vi "Plot_Server_Data.vi"() -> ()   [LabVIEW 2016]
uses:
  Anemometry/Anemometry Sub Vis/Controls/Server_Comms.ctl
  Anemometry/Anemometry Sub Vis/File/Setup_Filetype.ctl
  Anemometry/Anemometry Sub Vis/Globals/Preference_global.vi
panel:
  out "LastUpdated":string="Tue, May 12, 2015 at 11:28"
  in  "Throwback\n(mins)":dbl format="%.1f"
  in  "stop":bool=TRUE
  in  "Mode":T1(ring)=enum."Display data over specified period:"
  in  "History\n(mins)":dbl=20.0 format="%.1f"
  in  "Save plot number":T2(ring)
  out "Plot 3 Chs":string[](array[string])
  out "Plot 2 Chs":string[](array[string])
  out "Plot 1 Chs":string[](array[string])
  in  "Selector 1":i32[](listbox)
  in  "Search 1":string caption="Search:"
  in  "Search 2":string caption="Search:"
  in  "Search 3":string caption="Search:"
  in  "Selector 3":i32[](listbox)
  in  "Selector 2":i32[](listbox)
  in  "Precision":i32=2
  in  "Save 3":bool
  in  "palette3":i32(ring)=5 caption="Palette" items=["Strong", "Dark", "Light", "Pastel", "Pale", "Brash", "Clean", "Tidy"]
  out "Plot 3":cluster{"Times":dbl[], "Output array":dbl[]}[](graph)
  in  "Save 2":bool
  in  "palette2":i32(ring)=5 caption="Palette" items=["Strong", "Dark", "Light", "Pastel", "Pale", "Brash", "Clean", "Tidy"]
  out "Plot 2":cluster{"Times":dbl[], "Output array":dbl[]}[](graph)
  in  "Save 1":bool
  in  "palette1":i32(ring)=5 caption="Palette" items=["Strong", "Dark", "Light", "Pastel", "Pale", "Brash", "Clean", "Tidy"]
  out "Plot 1":cluster{"Times":dbl[], "Output array":dbl[]}[](graph)
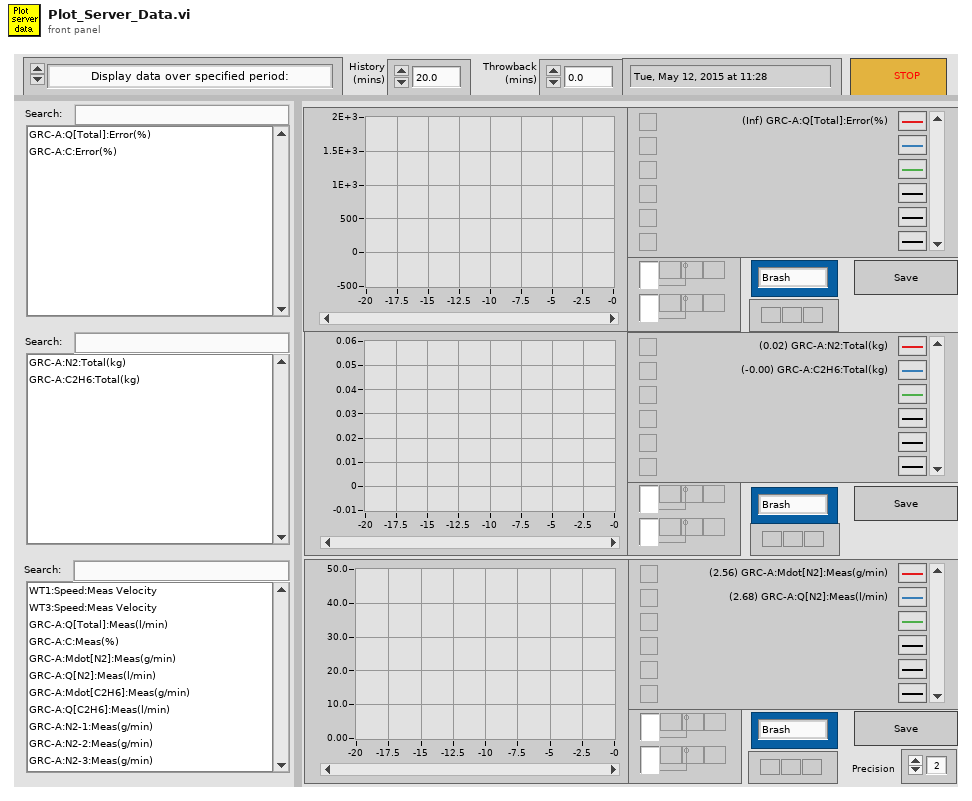
[diagram p1: front panel]
types:
  T1 = enum16{"Display full time history", "Display data over specified period:"}
  T2 = enum16{"Save Plot 1", "Save Plot 2", "Save Plot 3"}
  T3 = typedef "Server_Comms.ctl" = enum16{"Server Link Healthy", "Do Not Link To Server"}
  T4 = typedef "Setup_Filetype.ctl" = enum16{"Measurement Setups", "Calibration Setups", "General", "Results File Plotter Setups", "Speed Calib Tweaks"}
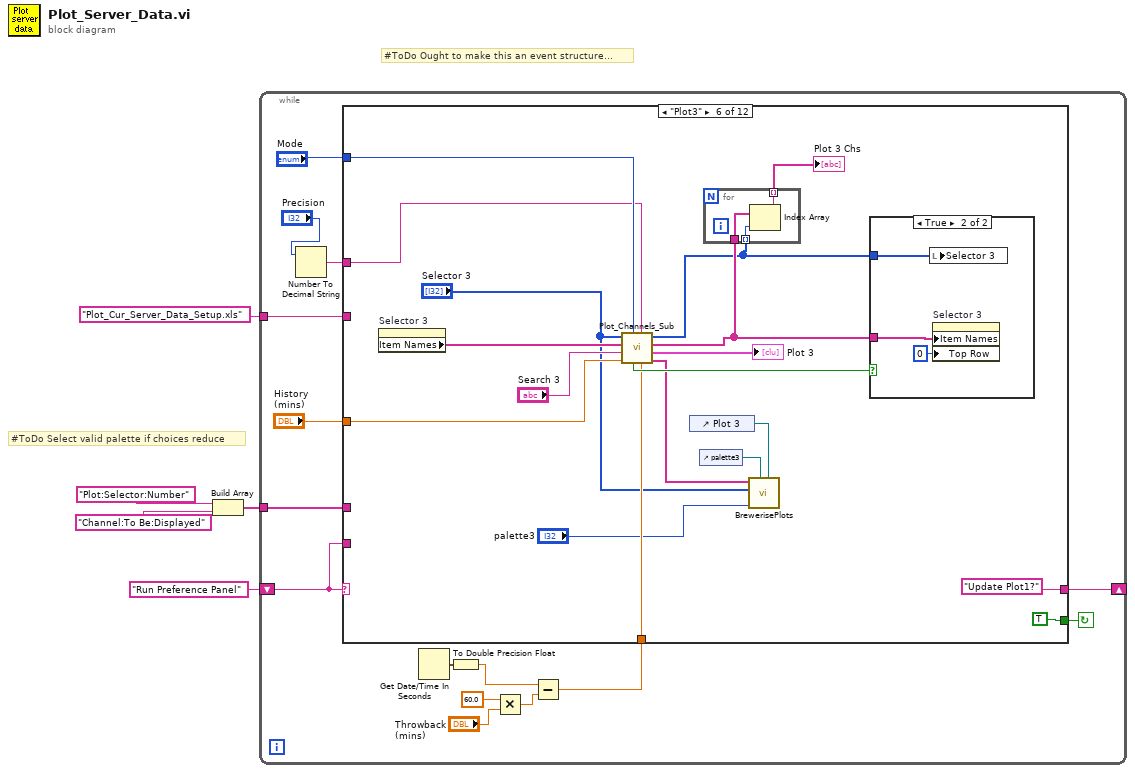
[diagram p0: block diagram]
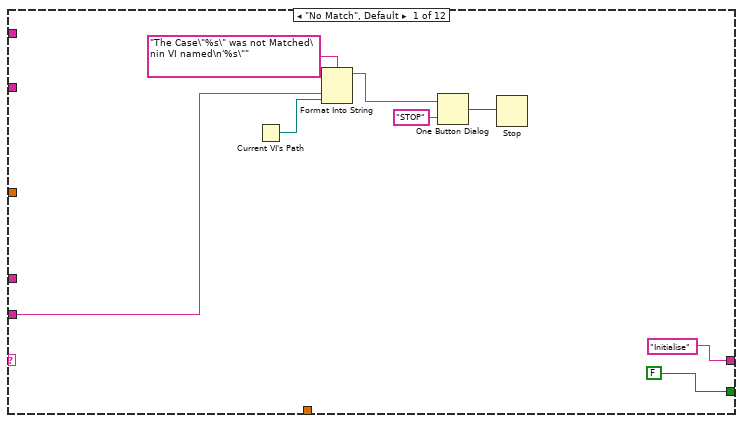
[diagram p2: hidden frame]
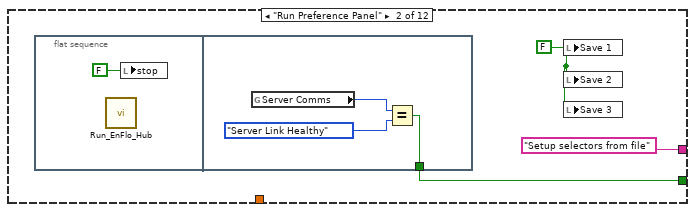
[diagram p3: hidden frame]
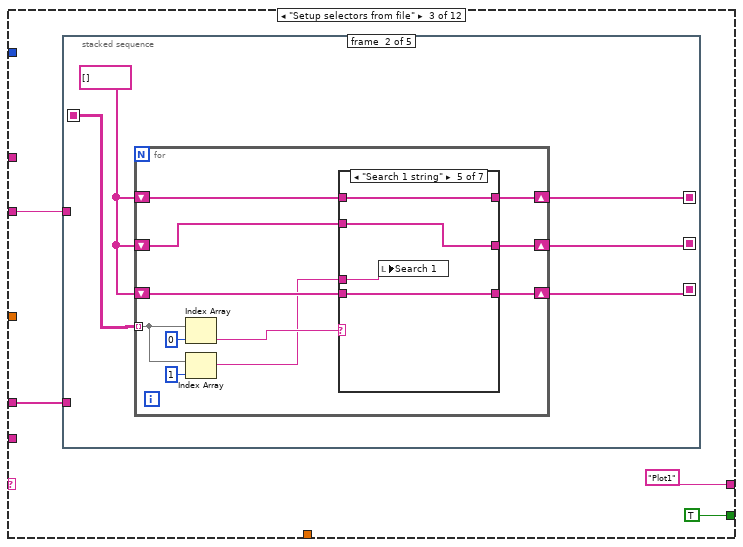
[diagram p4: hidden frame]
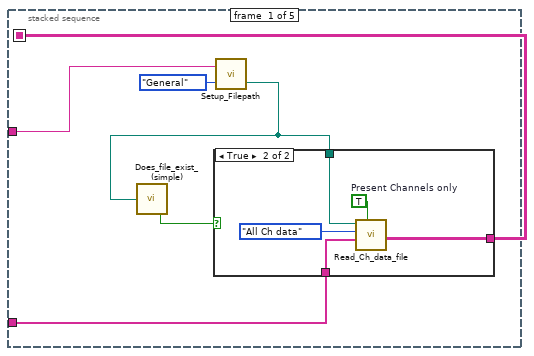
[diagram p5: hidden frame]
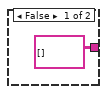
[diagram p6: hidden frame]
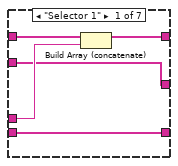
[diagram p7: hidden frame]
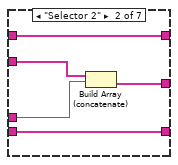
[diagram p8: hidden frame]
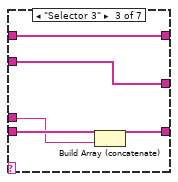
[diagram p9: hidden frame]
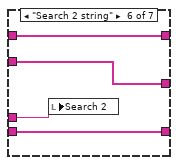
[diagram p11: hidden frame]
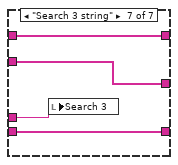
[diagram p12: hidden frame]
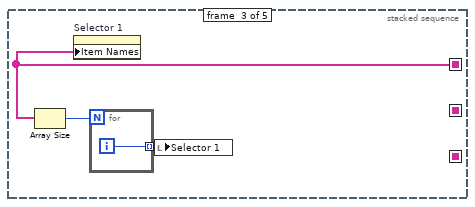
[diagram p13: hidden frame]
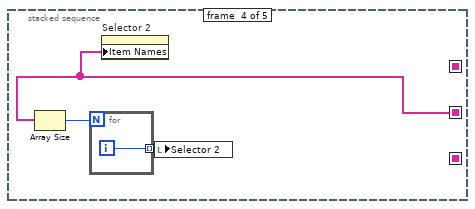
[diagram p14: hidden frame]
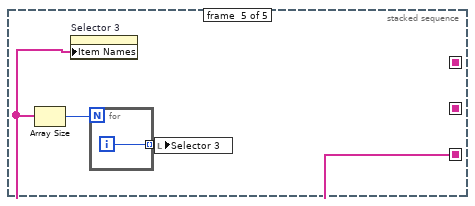
[diagram p15: hidden frame]
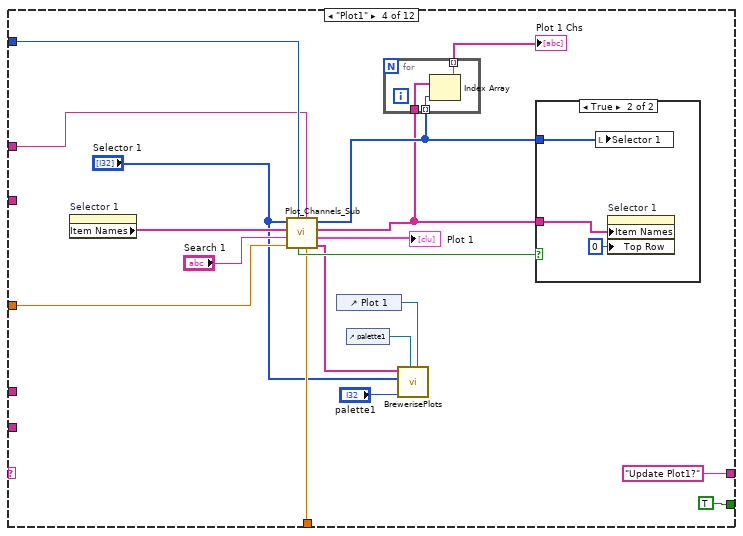
[diagram p16: hidden frame]
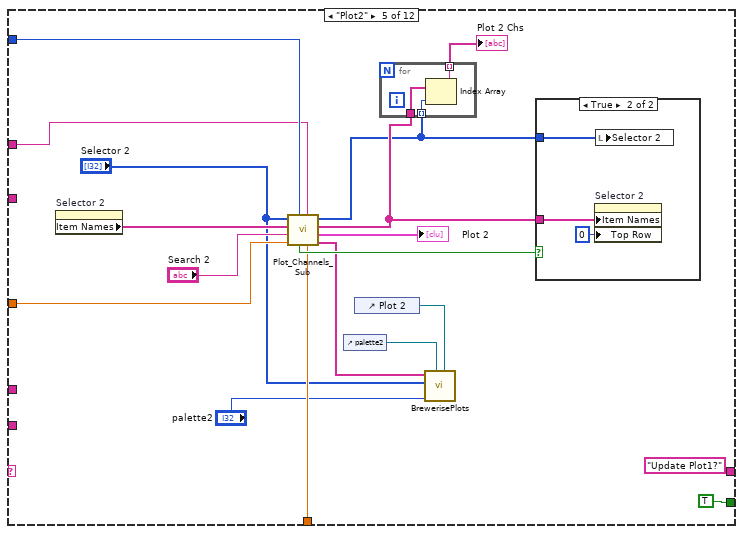
[diagram p18: hidden frame]
diagram:
  # "#ToDo Select valid palette if choices reduce"
  # "#ToDo Ought to make this an event structure..."
  n1 = Build Array("Plot:Selector:Number", "Channel:To Be:Displayed") -> (w2:string[])
  n2 = while {
    shift-left: "Run Preference Panel" -> [w18]
    shift-right: [w19] -> _
    tunnel: w2 -> [w15]
    tunnel: "Plot_Cur_Server_Data_Setup.xls" -> [w14]
    stop <- w20 continue-if-true
    n3 = Number To Decimal String(number="Precision") -> (decimal integer string=w12:string)  [unwired: 1 out]
    n4 = Get Date/Time In Seconds() -> (seconds since 1Jan1904=w11:timestamp)
    n5 = To Double Precision Float(number=w11) -> (double precision float=w7:dbl)
    n6 = Multiply(x=60.0, y="Throwback\n(mins)") -> (x*y=w8:dbl)
    n7 = Subtract(x=w7, y=w8) -> (x-y=w6:dbl)
    n8 = case shown="\"Plot3\"" w18 {
      tunnel: [FALSE w30 TRUE TRUE TRUE TRUE TRUE TRUE TRUE TRUE w323 w388] -> w20
      tunnel: ["Initialise" "Setup selectors from file" "Plot1" "Update Plot1?" "Update Plot1?" "Update Plot1?" w186 w212 w237 w271 w324 "Update Plot1?" ("t")] -> w19
      tunnel: w18 -> [w23 _ _ _ _ _ _ _ _ _ _ _]
      tunnel: "Mode" -> [_ _ _ w121 w148 w172 _ _ _ _ _ _]
      tunnel: "History\n(mins)" -> [_ _ _ w120 w147 w171 _ _ _ _ _ _]
      tunnel: w15 -> [_ _ w36 _ _ _ _ _ _ _ _ w392]
      tunnel: w14 -> [_ _ w37 _ _ _ _ _ _ _ _ w391]
      tunnel: w12 -> [_ _ _ w116 w140 w164 _ _ _ _ _ _]
      tunnel: w6 -> [_ _ _ w115 w139 w163 _ _ _ _ _ _]
      frame "No Match", Default {
        n9 = Current VI's Path() -> (path=w22:path)
        n10 = Format Into String(format string="The Case\"%s\" was not Matched\nin VI named\n'%s\"" ("Format String"), w23, w22) -> (resulting string=w26:string)  [unwired: 2 in, 1 out]
        n11 = One Button Dialog(message=w26, button name ("OK")="STOP") -> (true=w24:bool)
        n12 = Stop(stop? (T)=w24) -> ()
      }
      frame "Run Preference Panel" {
        w29 = FALSE ("Save 1")
        n13 = flat-sequence {
          tunnel: [w33] -> w30
          frame #0 {
            n14 = call "Run_EnFlo_Hub.vi"() -> ()  [unwired: 1 in, 7 out]
            n15 = local write "stop"(FALSE ("stop")) -> ()
          }
          frame #1 {
            n16 = global read "Preference_global.vi" "Server Comms"() -> (w34:T3)
            n17 = Equal?(x=w34, y=Server_Comms."Server Link Healthy" ("Server Comms")) -> (x = y?=w33:bool)
          }
        }
        n18 = local write "Save 1"(w29) -> ()
        n19 = local write "Save 2"(w29) -> ()
        n20 = local write "Save 3"(w29) -> ()
      }
      frame "Setup selectors from file" {
        n21 = stacked-sequence {
          seq-local: [w43 _ _ _ _] -> [_ w56 _ _ _]
          seq-local: [_ w54 _ _ _] -> [_ _ w100 _ _]
          seq-local: [_ w52 _ _ _] -> [_ _ _ w102 _]
          seq-local: [_ w53 _ _ _] -> [_ _ _ _ w106]
          tunnel: w37 -> [w42 _ _ _ _]
          tunnel: w36 -> [w44 _ _ _ _]
          frame #0 {
            n22 = call "Setup_Filepath.vi"("Setup File Type"=Setup_Filetype."General", "Filename in"=w42) -> ("Filename Out"=w41:path)  [unwired: 1 out]
            n23 = call "Does_file_exist_(simple).vi"("Pathname"=w41) -> ("exists?"=w45:bool)
            n24 = case shown="True" w45 {
              tunnel: w41 -> [_ w51]
              tunnel: w44 -> [_ w50]
              tunnel: [string[][] [] ("Channel Values") w47] -> w43
              frame False {
              }
              frame True {
                w49 = TRUE  # Present Channels only
                n25 = call "Read_Ch_data_file.vi"("Present Channels only"=w49, "Present Channels"=w50, "Output"=enum16{"All Ch data", "The last few rows"}."All Ch data", "Filename"=w51) -> ("Channel Values"=w47:string[][])  [unwired: 1 in, 4 out]
              }
            }
          }
          frame #1 {
            w55 = string[] []
            n26 = for {
              shift-right: [w62] -> w54
              shift-left: w55 -> [w63]
              tunnel: w56 -> [w64] mode=indexing
              shift-right: [w60] -> w52
              shift-left: w55 -> [w61]
              shift-right: [w58] -> w53
              shift-left: w55 -> [w59]
              n27 = Index Array(array=w64, index=0 ("Index")) -> (element=w66:string)
              n28 = Index Array(array=w64, index=1 ("Index")) -> (element=w57:string)
              n29 = case shown="\"Search 1 string\"" w66 {
                tunnel: w63 -> [w72 w77 w78 w84 w88 w92 w96]
                tunnel: [w71 w77 w78 w84 w88 w92 w96] -> w62
                tunnel: w57 -> [w70 w74 w80 _ w86 w90 w94]
                tunnel: w61 -> [w69 w75 w79 w85 w89 w93 w97]
                tunnel: [w69 w73 w79 w85 w89 w93 w97] -> w60
                tunnel: w59 -> [w68 w76 w82 w83 w87 w91 w95]
                tunnel: [w68 w76 w81 w83 w87 w91 w95] -> w58
                frame "Selector 1" {
                  n30 = Build Array (concatenate)(w72, w70) -> (w71:string[])
                }
                frame "Selector 2" {
                  n31 = Build Array (concatenate)(w75, w74) -> (w73:string[])
                }
                frame "Selector 3" {
                  n32 = Build Array (concatenate)(w82, w80) -> (w81:string[])
                }
                frame "No Match", Default {
                }
                frame "Search 1 string" {
                  n33 = local write "Search 1"(w86) -> ()
                }
                frame "Search 2 string" {
                  n34 = local write "Search 2"(w90) -> ()
                }
                frame "Search 3 string" {
                  n35 = local write "Search 3"(w94) -> ()
                }
              }
            }
          }
          frame #2 {
            n36 = Array Size(array=w100) -> (size(s)=w99:i32)
            n37 = property on="Selector 1" class="LstBox (strict)"("Item Names"=w100) -> ()  [unwired: 2 in, 2 out]
            n38 = for {
              N: w99 -> [_]
              tunnel: [w101] -> w98 mode=indexing
              i -> [w101]
            }
            n39 = local write "Selector 1"(w98) -> ()
          }
          frame #3 {
            n40 = Array Size(array=w102) -> (size(s)=w104:i32)
            n41 = for {
              N: w104 -> [_]
              tunnel: [w105] -> w103 mode=indexing
              i -> [w105]
            }
            n42 = property on="Selector 2" class="LstBox (strict)"("Item Names"=w102) -> ()  [unwired: 2 in, 2 out]
            n43 = local write "Selector 2"(w103) -> ()
          }
          frame #4 {
            n44 = Array Size(array=w106) -> (size(s)=w108:i32)
            n45 = property on="Selector 3" class="LstBox (strict)"("Item Names"=w106) -> ()  [unwired: 2 in, 2 out]
            n46 = for {
              N: w108 -> [_]
              tunnel: [w109] -> w107 mode=indexing
              i -> [w109]
            }
            n47 = local write "Selector 3"(w107) -> ()
          }
        }
      }
      frame "Plot1" {
        n48 = property on="Selector 1" class="LstBox (strict)"() -> ("Item Names"=w122:string[])  [unwired: 2 in, 2 out]
        n49 = call "Plot_Channels_Sub.vi"("End Time"=w115, "precision"=w116, "Mode"=w121, "History (min)"=w120, "Search String"="Search 1", "Selector List In"=w122, "Selector array In"="Selector 1") -> ("Plot Legend"=w112:string[], "Plot"=→"Plot 1":cluster{"Times":dbl[], "Output array":dbl[]}[], "Selector List Out"=w118:string[], "Selector array Out"=w119:i32[], "Selector Changed?"=w124:bool)
        n50 = control-ref of="Plot 1"() -> (w114:refnum<vi>)
        n51 = control-ref of="palette1"() -> (w113:refnum<vi>)
        n52 = for {
          tunnel: w119 -> [w130] mode=indexing
          tunnel: w118 -> [w129]
          tunnel: [w128] -> w117 mode=indexing
          n53 = Index Array(array=w129, index=w130) -> (element=w128:string)
        }
        "Plot 1 Chs" <- w117
        n54 = call "BrewerisePlots.vi"("graphRefnum"=w114, "paletteRefnum"=w113, "paletteNum"="palette1", "Series"="Selector 1", "Plot Legends"=w112) -> ()  [unwired: 7 in]
        n55 = case shown="True" w124 {
          tunnel: w118 -> [_ w133]
          tunnel: w119 -> [_ w132]
          frame False {
          }
          frame True {
            n56 = local write "Selector 1"(w132) -> ()
            n57 = property on="Selector 1" class="LstBox (strict)"("Item Names"=w133, "Top Row"=0) -> ()  [unwired: 2 in, 2 out]
          }
        }
      }
      frame "Plot2" {
        n58 = property on="Selector 2" class="LstBox (strict)"() -> ("Item Names"=w144:string[])  [unwired: 2 in, 2 out]
        n59 = call "Plot_Channels_Sub.vi"("End Time"=w139, "precision"=w140, "Mode"=w148, "History (min)"=w147, "Search String"="Search 2", "Selector List In"=w144, "Selector array In"="Selector 2") -> ("Plot Legend"=w136:string[], "Plot"=→"Plot 2":cluster{"Times":dbl[], "Output array":dbl[]}[], "Selector List Out"=w143:string[], "Selector array Out"=w142:i32[], "Selector Changed?"=w149:bool)
        n60 = control-ref of="palette2"() -> (w137:refnum<vi>)
        n61 = control-ref of="Plot 2"() -> (w138:refnum<vi>)
        n62 = for {
          tunnel: w142 -> [w154] mode=indexing
          tunnel: w143 -> [w153]
          tunnel: [w152] -> w141 mode=indexing
          n63 = Index Array(array=w153, index=w154) -> (element=w152:string)
        }
        "Plot 2 Chs" <- w141
        n64 = call "BrewerisePlots.vi"("graphRefnum"=w138, "paletteRefnum"=w137, "paletteNum"="palette2", "Series"="Selector 2", "Plot Legends"=w136) -> ()  [unwired: 7 in]
        n65 = case shown="True" w149 {
          tunnel: w143 -> [_ w156]
          tunnel: w142 -> [_ w157]
          frame False {
          }
          frame True {
            n66 = property on="Selector 2" class="LstBox (strict)"("Item Names"=w156, "Top Row"=0) -> ()  [unwired: 2 in, 2 out]
            n67 = local write "Selector 2"(w157) -> ()
          }
        }
      }
      frame "Plot3" {
        n68 = property on="Selector 3" class="LstBox (strict)"() -> ("Item Names"=w168:string[])  [unwired: 2 in, 2 out]
        n69 = call "Plot_Channels_Sub.vi"("End Time"=w163, "precision"=w164, "Mode"=w172, "History (min)"=w171, "Search String"="Search 3", "Selector List In"=w168, "Selector array In"="Selector 3") -> ("Plot Legend"=w160:string[], "Plot"=→"Plot 3":cluster{"Times":dbl[], "Output array":dbl[]}[], "Selector List Out"=w167:string[], "Selector array Out"=w166:i32[], "Selector Changed?"=w173:bool)
        n70 = control-ref of="Plot 3"() -> (w162:refnum<vi>)
        n71 = control-ref of="palette3"() -> (w161:refnum<vi>)
        n72 = for {
          tunnel: w166 -> [w178] mode=indexing
          tunnel: w167 -> [w177]
          tunnel: [w176] -> w165 mode=indexing
          n73 = Index Array(array=w177, index=w178) -> (element=w176:string)
        }
        "Plot 3 Chs" <- w165
        n74 = call "BrewerisePlots.vi"("graphRefnum"=w162, "paletteRefnum"=w161, "paletteNum"="palette3", "Series"="Selector 3", "Plot Legends"=w160) -> ()  [unwired: 7 in]
        n75 = case shown="True" w173 {
          tunnel: w167 -> [_ w180]
          tunnel: w166 -> [_ w181]
          frame False {
          }
          frame True {
            n76 = local write "Selector 3"(w181) -> ()
            n77 = property on="Selector 3" class="LstBox (strict)"("Item Names"=w180, "Top Row"=0) -> ()  [unwired: 2 in, 2 out]
          }
        }
      }
      frame "Update Plot1?" {
        n78 = while {
          shift-right: [w206] -> w193
          shift-left: _ -> [w203]
          shift-right: [w205] -> w195
          shift-left: _ -> [w204]
          tunnel: [w204] -> w194
          tunnel: [w203] -> w192
          shift-right: [w201] -> w183
          shift-left: _ -> [w200]
          tunnel: [w200] -> w184
          stop <- FALSE continue-if-true
          n79 = local read "Selector 1"() -> (w206:i32[])
          n80 = local read "palette1"() -> (w201:i32)
          n81 = local read "Search 1"() -> (w205:string)
        }
        n82 = case shown="False" "Save 1" {
          tunnel: ["Update Plot2?" "Save Plot" ("t")] -> w185
          frame False {
          }
          frame True {
            n83 = local write "Save plot number"(T2."Save Plot 1" ("Save plot number")) -> ()
          }
        }
        n84 = Equal?(x=w183, y=w184) -> (x = y?=w182:bool)
        n85 = Equal?(x=w193, y=w192) -> (x = y?=w190:bool)
        n86 = Equal?(x=w194, y=w195) -> (x = y?=w191:bool)
        n87 = Compound Arithmetic op=AND(w182, w190, w191) -> (w189:bool)
        n88 = Select(t=w185, s=w189, f="Plot1") -> (s? t:f=w186:string)
      }
      frame "Update Plot2?" {
        n89 = while {
          shift-right: [w231] -> w218
          shift-left: _ -> [w228]
          shift-right: [w230] -> w220
          shift-left: _ -> [w229]
          tunnel: [w229] -> w219
          tunnel: [w228] -> w217
          shift-right: [w226] -> w208
          shift-left: _ -> [w225]
          tunnel: [w225] -> w209
          stop <- FALSE continue-if-true
          n90 = local read "Selector 2"() -> (w231:i32[])
          n91 = local read "Search 2"() -> (w230:string)
          n92 = local read "palette2"() -> (w226:i32)
        }
        n93 = case shown="False" "Save 2" {
          tunnel: ["Update Plot3?" "Save Plot" ("t")] -> w210
          frame False {
          }
          frame True {
            n94 = local write "Save plot number"(T2."Save Plot 2" ("Save plot number")) -> ()
          }
        }
        n95 = Equal?(x=w208, y=w209) -> (x = y?=w207:bool)
        n96 = Equal?(x=w218, y=w217) -> (x = y?=w215:bool)
        n97 = Equal?(x=w219, y=w220) -> (x = y?=w216:bool)
        n98 = Compound Arithmetic op=AND(w207, w215, w216) -> (w214:bool)
        n99 = Select(t=w210, s=w214, f="Plot2") -> (s? t:f=w212:string)
      }
      frame "Update Plot3?" {
        n100 = while {
          shift-right: [w256] -> w243
          shift-left: _ -> [w253]
          shift-right: [w255] -> w245
          shift-left: _ -> [w254]
          tunnel: [w254] -> w244
          tunnel: [w253] -> w242
          shift-right: [w251] -> w234
          shift-left: _ -> [w250]
          tunnel: [w250] -> w233
          stop <- FALSE continue-if-true
          n101 = local read "Selector 3"() -> (w256:i32[])
          n102 = local read "Search 3"() -> (w255:string)
          n103 = local read "palette3"() -> (w251:i32)
        }
        n104 = case shown="False" "Save 3" {
          tunnel: ["What to do next?" "Save Plot" ("t")] -> w235
          frame False {
          }
          frame True {
            n105 = local write "Save plot number"(T2."Save Plot 3" ("Save plot number")) -> ()
          }
        }
        n106 = Equal?(x=w243, y=w242) -> (x = y?=w240:bool)
        n107 = Equal?(x=w244, y=w245) -> (x = y?=w241:bool)
        n108 = Equal?(x=w234, y=w233) -> (x = y?=w232:bool)
        n109 = Compound Arithmetic op=AND(w232, w240, w241) -> (w239:bool)
        n110 = Select(t=w235, s=w239, f="Plot3") -> (s? t:f=w237:string)
      }
      frame "What to do next?" {
        n111 = Wait (ms)(milliseconds to wait=u32 300) -> ()  [unwired: 1 out]
        n112 = while {
          shift-right: [w287] -> _
          shift-left: _ -> [w286]
          shift-right: [w285] -> _
          shift-left: _ -> [w284]
          shift-right: [w277] -> _
          shift-left: _ -> [w276]
          tunnel: [w279] -> w270
          shift-right: [w273] -> w259
          shift-left: _ -> [w274]
          stop <- FALSE continue-if-true
          n113 = local read "History\n(mins)"() -> (w287:dbl)
          n114 = local read "Mode"() -> (w285:T1)
          n115 = Equal?(x=w287, y=w286) -> (x = y?=w283:bool)
          n116 = Equal?(x=w284, y=w285) -> (x = y?=w282:bool)
          n117 = And(x=w283, y=w282) -> (x .and. y?=w281:bool)
          n118 = Select(t=w276, s=w281, f=0) -> (s? t:f=w278:i32)
          n119 = case shown="0, Default" w278 {
            tunnel: ["Plot1" "Plot2" "Plot3" "Update Plot1?" "Update Plot1?" "Update Plot1?" "Update Plot1?"] -> w279
            tunnel: w278 -> [w290 w294 w298 w304 w310 w316 _]
            tunnel: [w289 w293 w297 w303 w309 w315 0] -> w277
            tunnel: w274 -> [w288 w292 w296 w301 w307 w312 w319]
            tunnel: [w288 w292 w296 w300 w306 w313 w318] -> w273
            frame 0, Default {
              n120 = Increment(x=w290) -> (x+1=w289:i32)
            }
            frame 1 {
              n121 = Increment(x=w294) -> (x+1=w293:i32)
            }
            frame 2 {
              n122 = Increment(x=w298) -> (x+1=w297:i32)
            }
            frame 3 {
              n123 = Add(x=w301, y=1) -> (x+y=w300:i32)
              n124 = Increment(x=w304) -> (x+1=w303:i32)
            }
            frame 4 {
              n125 = Add(x=w307, y=1) -> (x+y=w306:i32)
              n126 = Increment(x=w310) -> (x+1=w309:i32)
            }
            frame 5 {
              n127 = Add(x=w312, y=1) -> (x+y=w313:i32)
              n128 = Increment(x=w316) -> (x+1=w315:i32)
            }
            frame 6 {
              n129 = Add(x=w319, y=1) -> (x+y=w318:i32)
            }
          }
        }
        n130 = Get Date/Time String(date format (0)=enum16{"short", "long", "abbreviated"}."abbreviated") -> (date string=w266:string, time string=w267:string)  [unwired: 2 out]
        n131 = Concatenate Strings(w266, " at " ("Substring"), w267) -> (→"LastUpdated":string)
        n132 = Quotient & Remainder(x=w259, y=500) -> (x-y*floor(x/y)=w263:i32)  [unwired: 1 out]
        n133 = Equal To 0?(x=w263) -> (x = 0?=w261:bool)
        n134 = Or(x="stop", y=w261) -> (x .or. y?=w260:bool)
        n135 = Select(t="Save Channel Names", s=w260, f=w270) -> (s? t:f=w271:string)
      }
      frame "Save Plot" {
        n136 = stacked-sequence {
          seq-local: [w335 _] -> [_ w363]
          seq-local: [w330 _] -> [_ w365]
          seq-local: [w334 _] -> [_ w364]
          seq-local: [w325 _] -> [_ w353]
          tunnel: ["What to do next?" _] -> w324
          tunnel: [TRUE _] -> w323
          frame #0 {
            n137 = case shown="\"Save Plot 1\"" "Save plot number" {
              tunnel: [w343 w346 w349] -> w340
              tunnel: [w342 w345 w348] -> w335
              frame "Save Plot 1" {
                n138 = local read "Plot 1 Chs"() -> (w342:string[])
                n139 = local write "Save 1"(FALSE ("Save 1")) -> ()
                n140 = local read "Plot 1"() -> (w343:cluster{"Times":dbl[], "Output array":dbl[]}[])
              }
              frame "Save Plot 2" {
                n141 = local read "Plot 2 Chs"() -> (w345:string[])
                n142 = local write "Save 2"(FALSE ("Save 1")) -> ()
                n143 = local read "Plot 2"() -> (w346:cluster{"Times":dbl[], "Output array":dbl[]}[])
              }
              frame "Save Plot 3" {
                n144 = local read "Plot 3 Chs"() -> (w348:string[])
                n145 = local write "Save 3"(FALSE ("Save 1")) -> ()
                n146 = local read "Plot 3"() -> (w349:cluster{"Times":dbl[], "Output array":dbl[]}[])
              }
            }
            n147 = Index Array(array=w340, index=0) -> (element=w338:cluster{"Times":dbl[], "Output array":dbl[]})
            n148 = Unbundle(w338) -> ("Times"=w329:dbl[])  [unwired: 1 out]
            n149 = Get Date/Time In Seconds() -> (seconds since 1Jan1904=w332:timestamp)
            n150 = for {
              tunnel: w340 -> [w351] mode=indexing
              tunnel: [w350] -> w334 mode=indexing
              n151 = Unbundle(w351) -> ("Output array"=w350:dbl[])  [unwired: 1 out]
            }
            n152 = To Double Precision Float(number=w332) -> (double precision float=w331:dbl)
            n153 = Multiply(x=w329, y=60.0) -> (x*y=w327:dbl[])
            n154 = Add(x=w331, y=w327) -> (x+y=w330:dbl[])
            n155 = Index Array(array=w327) -> (element=w326:dbl)  [unwired: 1 in]
            n156 = Subtract(x=w327, y=w326) -> (x-y=w325:dbl[])
          }
          frame #1 {
            w358 = FALSE  # append to file? (new file:F)
            n157 = for {
              tunnel: w364 -> [w385]
              tunnel: w365 -> [w379] mode=indexing
              tunnel: [w381] -> w357 mode=indexing
              tunnel: w353 -> [w375] mode=indexing
              i -> [w384]
              n158 = Number To Decimal String(number=w379) -> (decimal integer string=w380:string)  [unwired: 1 out]
              n159 = Index Array(array=w385, index (col)=w384) -> (element=w383:dbl[])  [unwired: 1 in]
              n160 = Number To Fractional String(number=w375, precision (6)=i16 2) -> (F-format string=w374:string)  [unwired: 2 in]
              n161 = Get Date/Time String(seconds (now)=w379) -> (date string=w378:string, time string=w377:string)  [unwired: 2 out]
              n162 = for {
                tunnel: w383 -> [w387] mode=indexing
                tunnel: [w386] -> w382 mode=indexing
                n163 = call "Number_2_string.vi"("number"=w387) -> ("String"=w386:string)  [unwired: 1 in]
              }
              n164 = Build Array (concatenate)(w378, w377, w380, w374, w382) -> (w381:string[])
            }
            n165 = Build Array (concatenate)("Date::", "Centre:Time:", "Seconds:Since:1st Jan 1904", "Time:in:Seconds", w363) -> (w356:string[])
            n166 = call "Ch_names_to_rows.vi"("Channel Names"=w356) -> ("3 Row names"=w362:string[][])
            n167 = File Dialog(7:"Please choose file name" ("prompt")) -> (3:w370:path)  [unwired: 1 in, 8 out]
            n168 = Build Array (concatenate)(w362, w357) -> (w360:string[][])
            n169 = Strip Path(path=w370) -> (stripped path=w367:path, name=w369:string)
            n170 = call "Add_filename_suffix.vi"("Filename"=w369, "Suffix to add"=".xls") -> ("Filename out"=w366:string)  [unwired: 3 out]
            n171 = Array To Spreadsheet String(array=w360, 3:"%s" ("format string")) -> (spreadsheet string=w359:string)  [unwired: 1 out]
            n172 = Build Path(base path=w367, name or relative path=w366) -> (appended path=w355:path)
            n173 = call "Write_File_Simple.vi"("append to file? (new file:F)"=w358, "character string"=w359, "file path"=w355) -> ()  [unwired: 2 out]
          }
        }
      }
      frame "Save Channel Names" {
        n174 = stacked-sequence {
          seq-local: [w394 _ _] -> [_ w418 _]
          seq-local: [_ w417 _] -> [_ _ w431]
          tunnel: w392 -> [_ _ w432]
          tunnel: w391 -> [_ _ w429]
          frame #0 {
            n175 = for {
              N: 3 -> [_]
              shift-right: [w398] -> w394
              shift-left: string[][] [] -> [w400]
              i -> [w405]
              n176 = Increment(x=w405) -> (x+1=w402:i32)
              n177 = case shown="1, Default" w402 {
                tunnel: [w412 w413 w415] -> w404
                tunnel: [w411 w414 w416] -> w396
                frame 1, Default {
                  n178 = local read "Selector 1"() -> (w412:i32[])
                  n179 = property on="Selector 1" class="LstBox (strict)"() -> ("Item Names"=w411:string[])  [unwired: 2 in, 2 out]
                }
                frame 2 {
                  n180 = local read "Selector 2"() -> (w413:i32[])
                  n181 = property on="Selector 2" class="LstBox (strict)"() -> ("Item Names"=w414:string[])  [unwired: 2 in, 2 out]
                }
                frame 3 {
                  n182 = local read "Selector 3"() -> (w415:i32[])
                  n183 = property on="Selector 3" class="LstBox (strict)"() -> ("Item Names"=w416:string[])  [unwired: 2 in, 2 out]
                }
              }
              n184 = Format Into String(format string="%d" ("Format String"), initial string="Selector ", w402) -> (resulting string=w399:string)  [unwired: 1 in, 1 out]
              n185 = for {
                tunnel: w404 -> [w410] mode=indexing
                tunnel: w399 -> [w409]
                tunnel: [w407] -> w397 mode=indexing
                tunnel: w396 -> [w406]
                n186 = Index Array(array=w406, index=w410) -> (element=w408:string)
                n187 = Build Array(w409, w408) -> (w407:string[])
              }
              n188 = Build Array (concatenate)(w400, w397) -> (w398:string[][])
            }
          }
          frame #1 {
            n189 = local read "Search 1"() -> (w419:string)
            n190 = local read "Search 2"() -> (w420:string)
            n191 = local read "Search 3"() -> (w421:string)
            n192 = Build Array("Search 1 string" ("element"), w419) -> (w425:string[])
            n193 = Build Array("Search 3 string" ("element"), w421) -> (w427:string[])
            n194 = Build Array("Search 2 string" ("element"), w420) -> (w426:string[])
            n195 = Build Array (concatenate)(w418, w425, w426, w427) -> (w417:string[][])
          }
          frame #2 {
            n196 = call "Setup_Filepath.vi"("Setup File Type"=Setup_Filetype."General", "Filename in"=w429) -> ("Filename Out"=w428:path)  [unwired: 1 out]
            n197 = Array Size(array=w431) -> (size(s)=w435:i32[])
            n198 = Index Array(array=w435, index=1 ("Index")) -> (element=w434:i32)
            n199 = Not Equal To 0?(x=w434) -> (x != 0?=w433:bool)
            n200 = case shown="True" w433 {
              tunnel: w428 -> [w437 w442]
              tunnel: w431 -> [_ w443]
              tunnel: w432 -> [_ w444]
              frame False {
                n201 = Delete(path (use dialog)=w437) -> ()  [unwired: 1 in, 6 out]
              }
              frame True {
                w438 = FALSE  # append to file? (new file:F)
                n202 = call "Ch_names_to_rows.vi"("Channel Names"=w444) -> ("3 Row names"=w445:string[][])
                n203 = Build Array (concatenate)(w445, w443) -> (w440:string[][])
                n204 = Array To Spreadsheet String(array=w440, 3:"%s" ("format string")) -> (spreadsheet string=w439:string)  [unwired: 1 out]
                n205 = call "Write_File_Simple.vi"("append to file? (new file:F)"=w438, "character string"=w439, "file path"=w442) -> ()  [unwired: 2 out]
              }
            }
          }
        }
        n206 = local read "stop"() -> (w389:bool)
        n207 = Not(x=w389) -> (.not. x?=w388:bool)
      }
    }
  }
